vi "Read Stop When Parent Stopped.vi"(11 "TEMPLATE Actor in":refnum<class "TEMPLATE Actor.lvclass">) -> (2 "Stop When Parent Stopped":bool)   [LabVIEW 2025, in "_Template.lvlib" / "Templates.lvlib" / "TEMPLATE Actor.lvlib" / "TEMPLATE Actor.lvclass"]
uses:
  TEMPLATE Actor.lvclass
  TEMPLATE Actor.lvclass/TEMPLATE Actor.ctl
  jettl/jettl/Actor/Actor/Actor.lvclass
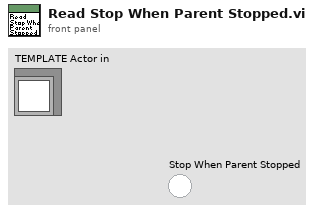
[diagram p1: front panel]
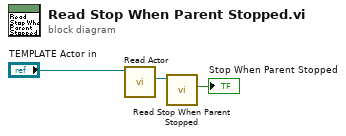
[diagram p0: block diagram]
diagram:
  n1 = call-dynamic "Read Actor.vi"("TEMPLATE Actor in"="TEMPLATE Actor in") -> ("Actor"=w2:refnum<class "Actor.lvclass">)  [unwired: 10 in]
  n2 = call-dynamic "Read Stop When Parent Stopped.vi"("Actor in"=w2) -> ("Stop When Parent Stopped"=→"Stop When Parent Stopped":bool)  [unwired: 10 in]
